vi "Rotate.vi"(8 "Area 2":dbl, 9 "Area 1":dbl, 10 "Center of Mass X2":dbl, 11 "Center of Mass X1":dbl) -> (1 "Area1- Area2 w/ deadband":dbl, 2 "Area 1 - Area 2 w/out deadband":dbl)   [LabVIEW 2014]
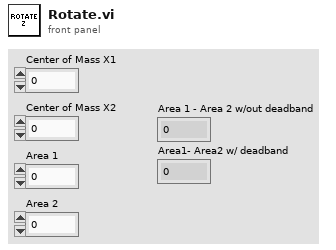
[diagram p1: front panel]
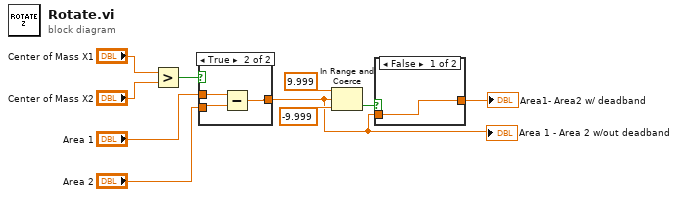
[diagram p0: block diagram]
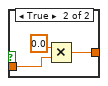
[diagram p2: hidden frame]
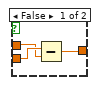
[diagram p3: hidden frame]
diagram:
  n1 = Greater?(x="Center of Mass X1", y="Center of Mass X2") -> (0:w8:bool)
  n2 = case shown="True" w8 {
    tunnel: "Area 1" -> [w12 w16]
    tunnel: "Area 2" -> [w13 w15]
    tunnel: [w11 w14] -> w2
    frame False {
      n3 = Subtract(x=w13, y=w12) -> (x-y=w11:dbl)
    }
    frame True {
      n4 = Subtract(x=w16, y=w15) -> (x-y=w14:dbl)
    }
  }
  "Area 1 - Area 2 w/out deadband" <- w2
  n5 = In Range and Coerce(upper limit=9.999, x=w2, lower limit=-9.999) -> (In Range?=w3:bool)  [unwired: 1 out]
  n6 = case shown="False" w3 {
    tunnel: w2 -> [w17 w19]
    tunnel: [w17 w18] -> w1
    frame False {
    }
    frame True {
      n7 = Multiply(x=0.0, y=w19) -> (x*y=w18:dbl)
    }
  }
  "Area1- Area2 w/ deadband" <- w1
